vi "Resistance Control.vi"() -> ()   [LabVIEW 2014]
uses:
  <vilib>/express/express arith-compare/Formula/XNode/ExpressFormulaBlockNode.xnode
panel:
  in  "Selector Switch":bool
  in  "?":bool
  in  "Watt User Input":dbl
  in  "Watts":dbl(slide) scale=3.0..6.9
  # "RL"
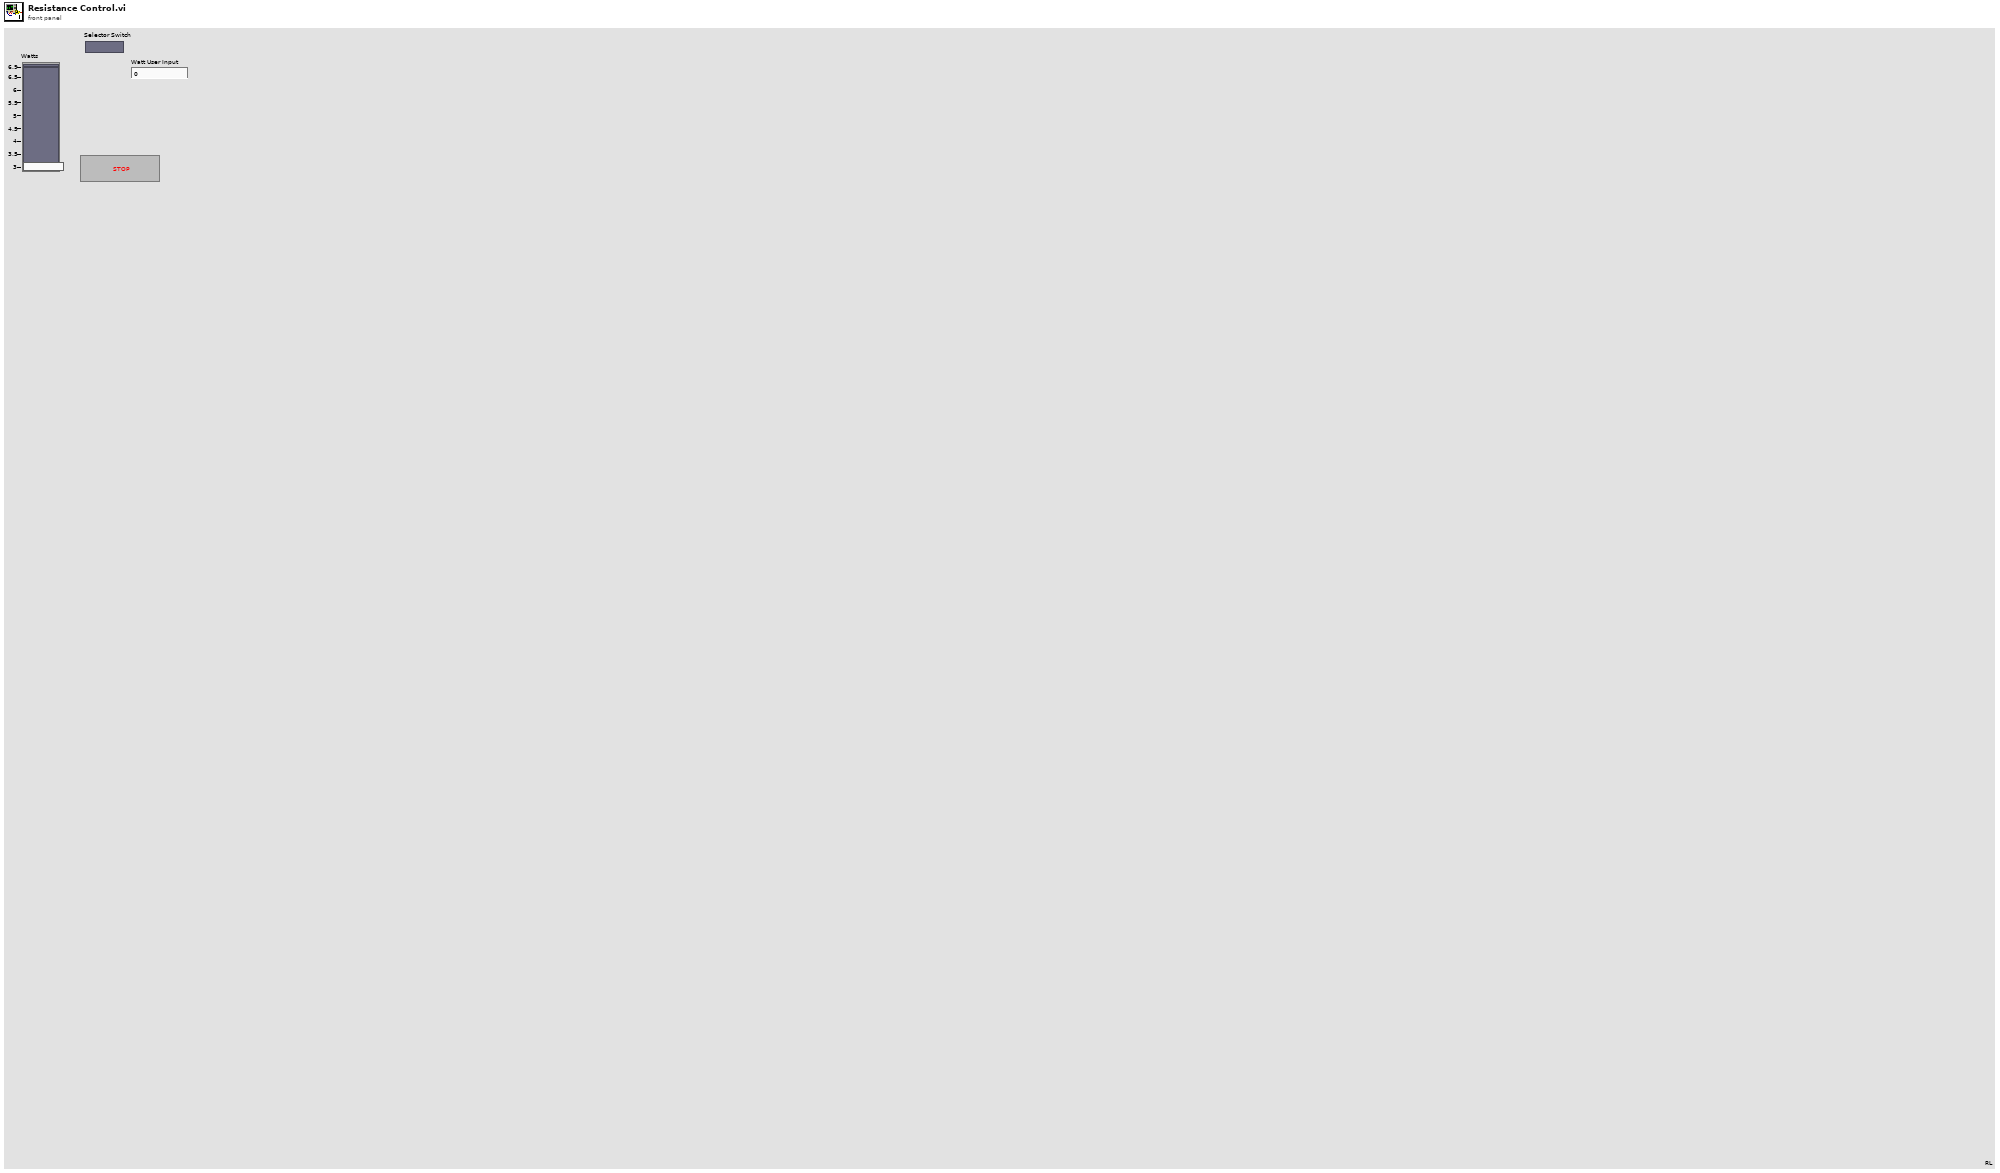
[diagram p1: front panel]
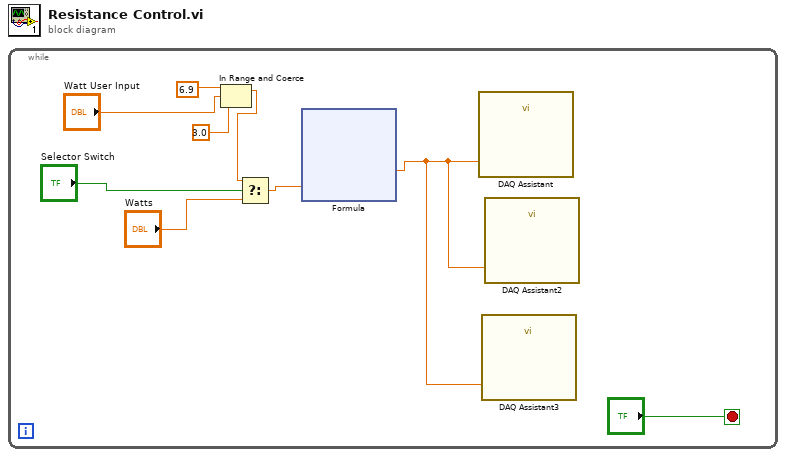
[diagram p0: block diagram]
diagram:
  n1 = while {
    stop <- "?" stop-if-true
    n2 = In Range and Coerce(upper limit=6.9, x="Watt User Input", lower limit=3.0) -> (coerced(x)=w5:dbl)  [unwired: 1 out]
    n3 = Select(t=w5, s="Selector Switch", f="Watts") -> (s? t:f=w6:dbl)
    n4 = xnode "Formula"("X"=w6) -> ("Result"=w2:dbl)  [unwired: 1 in, 1 out]
    n5 = call "DAQ Assistant"("data"=w2) -> ()  [unwired: 17 in, 2 out]
    n6 = call "DAQ Assistant3"("data"=w2) -> ()  [unwired: 17 in, 2 out]
    n7 = call "DAQ Assistant2"("data"=w2) -> ()  [unwired: 17 in, 2 out]
  }
